vi "Waveform_Size and Sync to End Time.vi"(10 "Size":i32, 11 "Waveform Out in":T1) -> (3 "Waveform Out out":T1)   [LabVIEW 2020]
uses:
  <vilib>/Waveform/WDTOps.llb/WDT Get Final Time Value DBL.vi
  Universal Controls/Waveform_Data.ctl
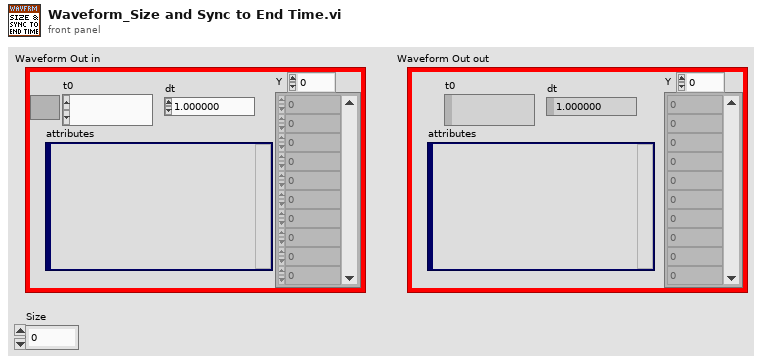
[diagram p1: front panel]
types:
  T1 = typedef "Waveform_Data.ctl" = waveform(dbl)
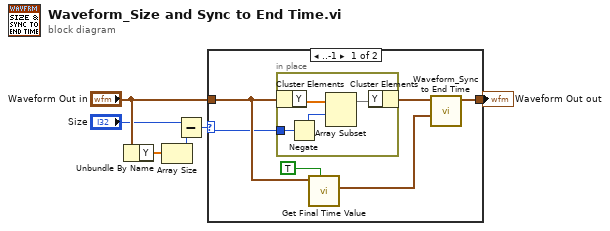
[diagram p0: block diagram]
diagram:
  n1 = Unbundle By Name("Waveform Out in") -> ("Y"=w1:dbl[])
  n2 = Array Size(array=w1) -> (size(s)=w2:i32)
  n3 = Subtract(x="Size", y=w2) -> (x-y=w4:i32)
  n4 = case shown="..-1" w4 {
    selector: w4 -> [w7 _]
    tunnel: "Waveform Out in" -> [w11 w17]
    tunnel: [w9 w17] -> w3
    frame ..-1 {
      n5 = in-place {
        in-place-border: w7 -> [w14]
        n6 = in-place-cluster #1(w11) -> ("Y"=w16:dbl[])
        n7 = Negate(x=w14) -> (-x=w13:i32)
        n8 = Array Subset(array=w16, index=w13) -> (w15:dbl[])  [unwired: 1 in]
        n9 = in-place-cluster #1("Y"=w15) -> (w10:T1)
      }
      n10 = call-poly <vilib>:"Get Final Time Value.vi"("open interval? (T)"=TRUE, "waveform in"=w11) -> ("tf"=w8:timestamp)  [unwired: 7 in, 2 out]
      n11 = call "Waveform_Sync to End Time.vi"("tf"=w8, "Waveform"=w10) -> ("Waveform Out"=w9:T1)  [unwired: 7 in, 2 out]
    }
    frame 0.. {
    }
  }
  "Waveform Out out" <- w3
